vi "MGI Daemon Implementation.vi"(9 "Ignore Warnings? (F: Process Errors and Warnings)":bool, 10 "Log Dir":path, 11 "MGI Error Reporter Dialog In":refnum<class "MGI Error Reporter Dialog.lvclass">) -> (3 "MGI Error Reporter Out":refnum<class "MGI Error Reporter Dialog.lvclass">)   [LabVIEW 2016, in "MGI Error Reporter Dialog.lvclass"]
doc: "Implementation of the Error Handler Loop. This VI is separated from the Front Panel Controls so that the front panel control VI could be overridden in a child class and the appearance changed.\n\nAuthored by Shawn Walpole\nsupport@mooregoodideas.com\nwww.mooregoodideas.com\n\nCopyright (c) 2013, Moore Good Ideas, Inc.\n\nAll rights reserved.\n\nRedistribution and use in source and binary forms, with or without modification, are permitted provided that the following conditions are met:\n\n * Redistributions of source code must retain the above copyright notice, this list of conditions and the following disclaimer.\n * Redistributions in binary form must reproduce the above copyright notice, this list of conditions and the following disclaimer in the documentation and/or other materials provided with the distribution.\n * Neither the name of Moore Good Ideas, Inc. nor the names of its contributors may be used to endorse or promote products derived from this software without specific prior written permission.\n\nTHIS SOFTWARE IS PROVIDED BY THE COPYRIGHT HOLDERS AND CONTRIBUTORS \"AS IS\" AND ANY EXPRESS OR IMPLIED WARRANTIES, INCLUDING, BUT NOT LIMITED TO, THE IMPLIED WARRANTIES OF MERCHANTABILITY AND FITNESS FOR A PARTICULAR PURPOSE ARE DISCLAIMED. IN NO EVENT SHALL THE COPYRIGHT OWNER OR CONTRIBUTORS BE LIABLE FOR ANY DIRECT, INDIRECT, INCIDENTAL, SPECIAL, EXEMPLARY, OR CONSEQUENTIAL DAMAGES (INCLUDING, BUT NOT LIMITED TO, PROCUREMENT OF SUBSTITUTE GOODS OR SERVICES; LOSS OF USE, DATA, OR PROFITS; OR BUSINESS INTERRUPTION) HOWEVER CAUSED AND ON ANY THEORY OF LIABILITY, WHETHER IN CONTRACT, STRICT LIABILITY, OR TORT (INCLUDING NEGLIGENCE OR OTHERWISE) ARISING IN ANY WAY OUT OF THE USE OF THIS SOFTWARE, EVEN IF ADVISED OF THE POSSIBILITY OF SUCH DAMAGE."
uses:
  <userlib>/_MGI/Error Reporter/MGI Error Reporter Dialog/MGI Error Reporter Dialog.lvclass
  <userlib>/_MGI/Error Reporter/MGI Error Reporter Dialog/MGI Error Reporter Dialog.lvclass/MGI Error Reporter Dialog.ctl
  <vilib>/event_ctls.llb/sizeaction.ctl
  <vilib>/event_ctls.llb/panelstate.ctl
  <userlib>/_MGI/Error Reporter/MGI Error Reporter Dialog/Protected/MGI Control Enum.ctl
  <userlib>/_MGI/Error Reporter/MGI Error Reporter Dialog/MGI ERD LB Row Base/MGI ERD LB Row Base.lvclass
  <userlib>/_MGI/Error Reporter/MGI Error Reporter Base/MGI Error Reporter Base.lvclass
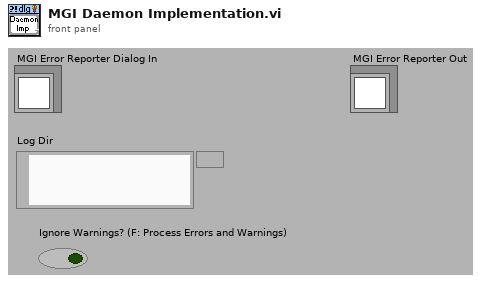
[diagram p1: front panel]
types:
  T1 = typedef "panelstate.ctl" = enum32{"Standard", "Minimized", "Maximized"}
  T2 = typedef "sizeaction.ctl" = enum32{"Minimized", "Maximized", "Resized"}
  T3 = typedef "LVRectTypeDef.ctl" = cluster{"Left":i16, "Top":i16, "Right":i16, "Bottom":i16}
  T4 = typedef "MGI Error Reporter Dialog.lvclass/MGI Control Enum.ctl" = enum16{"Error LB", "Details String", "Caller Ring", "Message String", "Clear Button"}
  T5 = typedef "LVPoint32TypeDef.ctl" = cluster{"Horizontal":i32, "Vertical":i32}
  T6 = typedef "MGI Error Reporter Dialog.lvclass/MGI Dialog UI Refs Cluster.ctl" = cluster{"LB Ref":refnum<vi>, "Details Ref":refnum<vi>, "Caller Ring Ref":refnum<vi>, "Message Ref":refnum<vi>, "Clear Btn Ref":refnum<vi>}
  T7 = typedef "MGI Error Reporter Base.lvclass/Cmd Enum.ctl" = enum16{"Quit", "Show UI"}
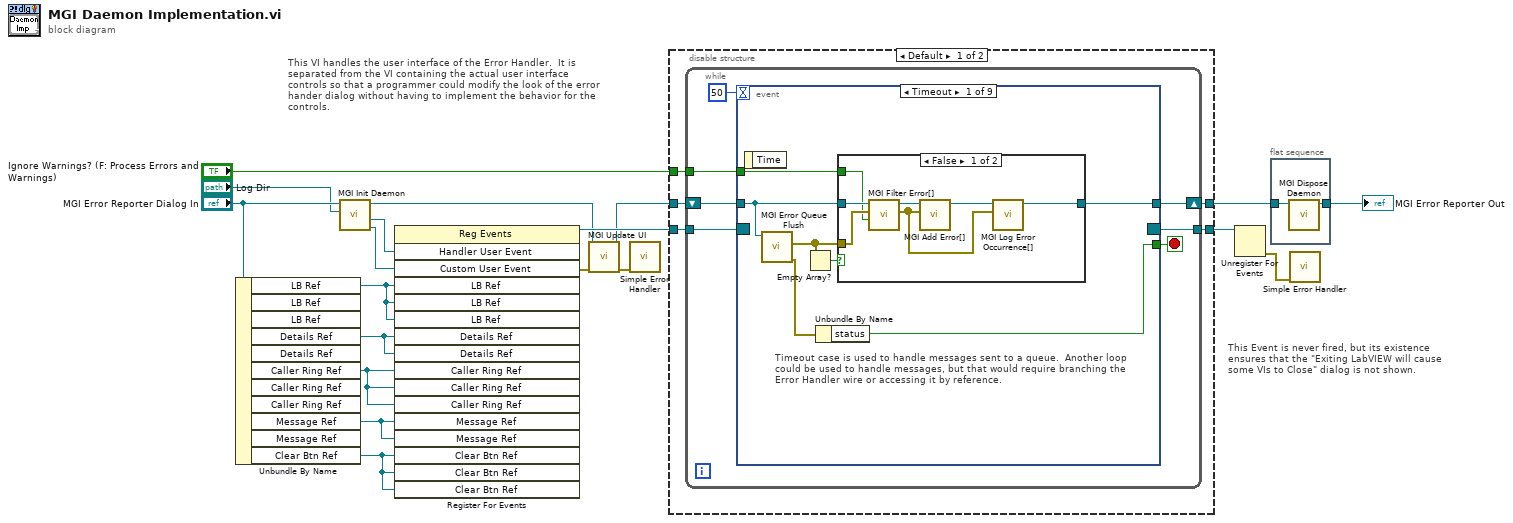
[diagram p0: block diagram]
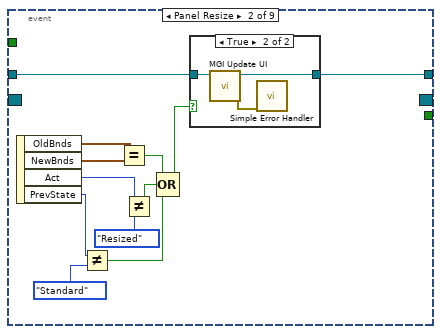
[diagram p3: hidden frame]
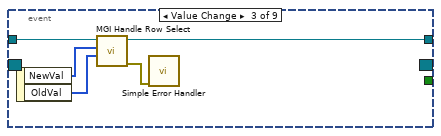
[diagram p5: hidden frame]
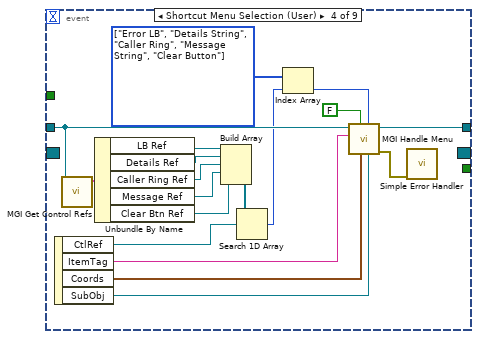
[diagram p6: hidden frame]
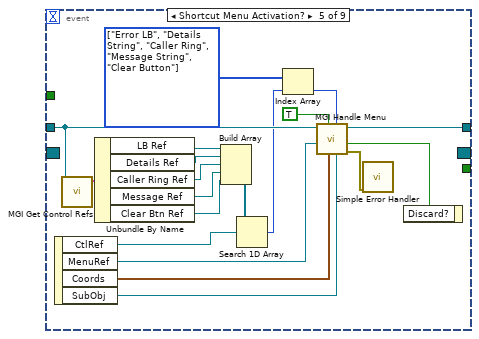
[diagram p7: hidden frame]
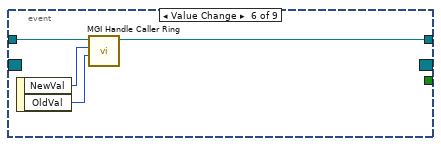
[diagram p8: hidden frame]
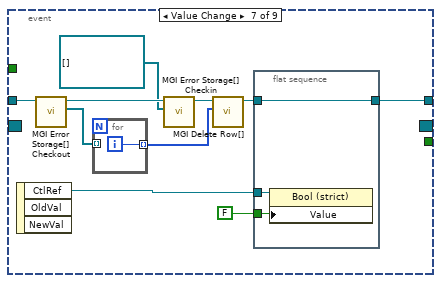
[diagram p9: hidden frame]
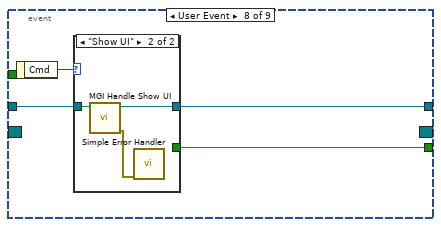
[diagram p10: hidden frame]
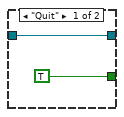
[diagram p11: hidden frame]
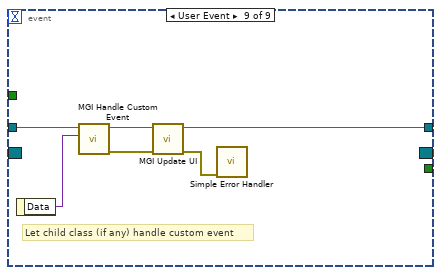
[diagram p12: hidden frame]
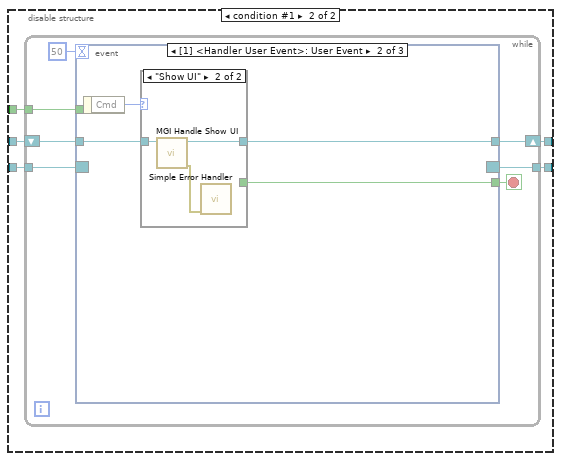
[diagram p13: hidden frame]
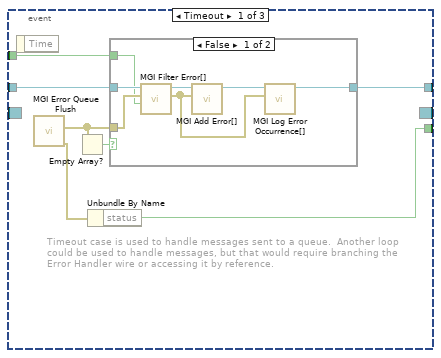
[diagram p14: hidden frame]
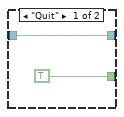
[diagram p16: hidden frame]
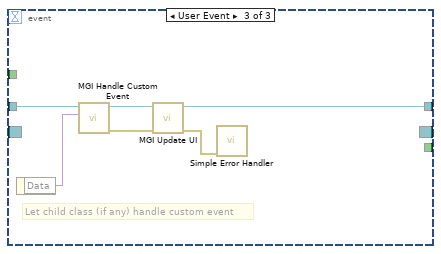
[diagram p17: hidden frame]
diagram:
  # "This Event is never fired, but its existence ensures that the \"Exiting LabVIEW will cause some VIs to Close\" dialog is not shown."
  # "This VI handles the user interface of the Error Handler.  It is separated from the VI containing the actual user interface controls so that a programmer could modify the look of the error hander dialog without having to implement the behavior for the controls."
  n1 = Unbundle By Name("MGI Error Reporter Dialog In") -> ("LB Ref"=w6:refnum<vi>, "Details Ref"=w5:refnum<vi>, "Caller Ring Ref"=w2:refnum<vi>, "Message Ref"=w8:refnum<vi>, "Clear Btn Ref"=w1:refnum<vi>)  [unwired: 6 out]
  n2 = call-dynamic "MGI Init Daemon.vi"("Err Dir"="Log Dir", "MGI Error Reporter Base In"="MGI Error Reporter Dialog In") -> ("Custom User Event"=w19:refnum<user-event>, "Handler User Event"=w18:refnum<user-event>, "MGI Error Reporter Base Out"=w11:refnum<class "MGI Error Reporter Dialog.lvclass">)  [unwired: 7 out]
  n3 = register-events(w18, w19, w6, w6, w6, w5, w5, w2, w2, w2, w8, w8, w1, w1, w1) -> (reference out=w17:refnum<event-registration>, error out=w13:errorcluster)  [unwired: 2 in]
  n4 = call-dynamic "MGI Update UI.vi"("error in (no error)"=w13, "MGI Error Handler in"=w11) -> ("error out"=w4:errorcluster, "MGI Error Handler out"=w14:refnum<class "MGI Error Reporter Dialog.lvclass">)  [unwired: 8 out]
  n5 = call <vilib>:"Simple Error Handler.vi"("error in (no error)"=w4) -> ()  [unwired: 1 in, 8 out]
  n6 = disable-structure shown="Default" {
    disable-tunnel: w17 -> [w24 w142]
    disable-tunnel: [w23 w141] -> w15
    disable-tunnel: w14 -> [w22 w140]
    disable-tunnel: [w21 w139] -> w12
    disable-tunnel: "Ignore Warnings? (F: Process Errors and Warnings)" -> [w20 w138]
    frame condition #0 (active) {
      n7 = while {
        tunnel: w24 -> [w25]
        shift-right: [w29] -> w23
        shift-left: w22 -> [w30]
        tunnel: [w27] -> w21
        tunnel: w20 -> [w26]
        stop <- w31 stop-if-true
        n8 = event shown="[0] Timeout" {
          selector: w25 -> [_ _ _ _ _ _ _ _ _]
          dyn-events: [_ _ _ _ _ _ _ _ _] -> w27
          timeout: 50 -> [_ _ _ _ _ _ _ _ _]
          tunnel: [w36 _ _ _ _ _ _ w123 _] -> w31
          tunnel: w30 -> [w32 w52 w67 w81 w101 w108 w113 w126 w137]
          tunnel: [w38 w51 w64 w79 w99 w107 w115 w125 w133] -> w29
          tunnel: w26 -> [w35 _ _ _ _ _ _ _ _]
          event Timeout {
            # "Timeout case is used to handle messages sent to a queue.  Another loop could be used to handle messages, but that would require branching the Error Handler wire or accessing it by reference."
            n9 = event-data() -> ()  [unwired: 2 out]
            n10 = call-dynamic "MGI Error Queue Flush.vi"("MGI Error Reporter Base In"=w32) -> ("error out"=w34:errorcluster, "Error[]"=w33:errorcluster[])  [unwired: 1 in, 8 out]
            n11 = Empty Array?(array=w33) -> (empty?=w37:bool)
            n12 = Unbundle By Name(w34) -> ("status"=w36:bool)
            n13 = case shown="False" w37 {
              tunnel: w32 -> [w44 w46]
              tunnel: [w39 w46] -> w38
              tunnel: w33 -> [w45 _]
              tunnel: w35 -> [w42 _]
              frame False {
                n14 = call-dynamic "MGI Filter Error[].vi"("Ignore Warnings? (F: Process Errors and Warnings)"=w42, "Error Occurence[]"=w45, "MGI Error Reporter Base in"=w44) -> ("Filtered Error[]"=w43:errorcluster[], "MGI Error Reporter Base out"=w41:refnum<class "MGI Error Reporter Dialog.lvclass">)  [unwired: 7 out]
                n15 = call-dynamic "MGI Add Error[].vi"("Error[]"=w43, "MGI Error Handler in"=w41) -> ("MGI Error Handler out"=w40:refnum<class "MGI Error Reporter Dialog.lvclass">)  [unwired: 1 in, 8 out]
                n16 = call-dynamic "MGI Log Error Occurrence[].vi"("Error Occurence[]"=w43, "MGI Error Reporter Base in"=w40) -> ("MGI Error Reporter Base out"=w39:refnum<class "MGI Error Reporter Dialog.lvclass">)  [unwired: 2 in, 7 out]
              }
              frame True {
              }
            }
          }
          event Panel Resize {
            n17 = event-data() -> ("OldBnds"=w58:T3, "NewBnds"=w57:T3, "Act"=w55:T2, "PrevState"=w49:T1)  [unwired: 1 out]
            n18 = Not Equal?(x=w49, y=panelstate."Standard" ("PrevState")) -> (x != y?=w47:bool)
            n19 = Equal?(x=w58, y=w57) -> (x = y?=w56:bool)
            n20 = Not Equal?(x=w55, y=sizeaction."Resized" ("Act")) -> (x != y?=w53:bool)
            n21 = Compound Arithmetic op=OR(w56, w53, w47) -> (w50:bool)
            n22 = case shown="True" w50 {
              tunnel: w52 -> [w59 w62]
              tunnel: [w59 w61] -> w51
              frame False {
              }
              frame True {
                n23 = call-dynamic "MGI Update UI.vi"("MGI Error Handler in"=w62) -> ("error out"=w60:errorcluster, "MGI Error Handler out"=w61:refnum<class "MGI Error Reporter Dialog.lvclass">)  [unwired: 1 in, 8 out]
                n24 = call <vilib>:"Simple Error Handler.vi"("error in (no error)"=w60) -> ()  [unwired: 1 in, 8 out]
              }
            }
          }
          event Value Change {
            n25 = event-data() -> ("NewVal"=w66:i32[], "OldVal"=w65:i32[])  [unwired: 1 out]
            n26 = call-dynamic "MGI Handle Row Select.vi"("Old Selected[]"=w65, "Selected[]"=w66, "MGI Error Handler in"=w67) -> ("error out"=w63:errorcluster, "MGI Error Handler out"=w64:refnum<class "MGI Error Reporter Dialog.lvclass">)  [unwired: 1 in, 6 out]
            n27 = call <vilib>:"Simple Error Handler.vi"("error in (no error)"=w63) -> ()  [unwired: 1 in, 8 out]
          }
          event Shortcut Menu Selection (User) {
            w72 = T4[] [enum."Error LB", enum."Details String", enum."Caller Ring", enum."Message String", enum."Clear Button"] items=["Error LB", "Details String", "Caller Ring", "Message String", "Clear Button"]
            n28 = event-data() -> ("CtlRef"=w73:refnum<vi>, "ItemTag"=w85:string, "Coords"=w83:T5, "SubObj"=w82:refnum<vi>)  [unwired: 1 out]
            n29 = call <userlib>:"MGI Get Control Refs.vi"("MGI Error Dialog.lvclass"=w81) -> ("Refs"=w80:T6)  [unwired: 10 out]
            n30 = Unbundle By Name(w80) -> ("LB Ref"=w78:refnum<vi>, "Details Ref"=w77:refnum<vi>, "Caller Ring Ref"=w76:refnum<vi>, "Message Ref"=w75:refnum<vi>, "Clear Btn Ref"=w68:refnum<vi>)
            n31 = Build Array(w78, w77, w76, w75, w68) -> (w74:refnum<vi>[])
            n32 = Search 1D Array(1D array=w74, element=w73) -> (index of element=w71:i32)  [unwired: 1 out]
            n33 = Index Array(array=w72, index=w71) -> (element=w70:T4)
            n34 = call-dynamic "MGI Handle Menu.vi"("SubObj"=w82, "Control Enum"=w70, "Coord"=w83, "Activation? (F:Selection)"=FALSE, "Selection:Menu Tag"=w85, "MGI Error Reporter Dialog"=w81) -> ("error out"=w69:errorcluster, "MGI Error Reporter Dialog Out"=w79:refnum<class "MGI Error Reporter Dialog.lvclass">)  [unwired: 2 in, 2 out]
            n35 = call <vilib>:"Simple Error Handler.vi"("error in (no error)"=w69) -> ()  [unwired: 1 in, 8 out]
          }
          event Shortcut Menu Activation? {
            w92 = T4[] [enum."Error LB", enum."Details String", enum."Caller Ring", enum."Message String", enum."Clear Button"] items=["Error LB", "Details String", "Caller Ring", "Message String", "Clear Button"]
            n36 = event-data() -> ("CtlRef"=w93:refnum<vi>, "MenuRef"=w89:refnum<k9>, "Coords"=w103:T5, "SubObj"=w102:refnum<vi>)  [unwired: 1 out]
            n37 = call <userlib>:"MGI Get Control Refs.vi"("MGI Error Dialog.lvclass"=w101) -> ("Refs"=w100:T6)  [unwired: 10 out]
            n38 = Unbundle By Name(w100) -> ("LB Ref"=w98:refnum<vi>, "Details Ref"=w97:refnum<vi>, "Caller Ring Ref"=w96:refnum<vi>, "Message Ref"=w95:refnum<vi>, "Clear Btn Ref"=w86:refnum<vi>)
            n39 = Build Array(w98, w97, w96, w95, w86) -> (w94:refnum<vi>[])
            n40 = Search 1D Array(1D array=w94, element=w93) -> (index of element=w91:i32)  [unwired: 1 out]
            n41 = Index Array(array=w92, index=w91) -> (element=w90:T4)
            n42 = call-dynamic "MGI Handle Menu.vi"("SubObj"=w102, "Control Enum"=w90, "Coord"=w103, "Activation? (F:Selection)"=TRUE, "Activation:MenuRef"=w89, "MGI Error Reporter Dialog"=w101) -> ("error out"=w87:errorcluster, "Activation:Discard?"=w88:bool, "MGI Error Reporter Dialog Out"=w99:refnum<class "MGI Error Reporter Dialog.lvclass">)  [unwired: 2 in, 1 out]
            n43 = call <vilib>:"Simple Error Handler.vi"("error in (no error)"=w87) -> ()  [unwired: 1 in, 8 out]
            n44 = event-data("Discard?"=w88) -> ()  [unwired: 1 in, 1 out]
          }
          event Value Change {
            n45 = event-data() -> ("NewVal"=w106:u16, "OldVal"=w105:u16)  [unwired: 1 out]
            n46 = call-dynamic "MGI Handle Caller Ring.vi"("Old Value"=w105, "New Value"=w106, "MGI Error Reporter Dialog in"=w108) -> ("MGI Error Reporter Dialog out"=w107:refnum<class "MGI Error Reporter Dialog.lvclass">)  [unwired: 1 in, 7 out]
          }
          event Value Change {
            n47 = event-data() -> ("CtlRef"=w117:refnum<vi>)  [unwired: 3 out]
            n48 = call <userlib>:"MGI Error Storage[] Checkout.vi"("MGI Error Reporter Dialog In"=w113) -> ("ErrStorage[row]"=w112:refnum<class "MGI ERD LB Row Base.lvclass">[], "MGI Error Reporter Dialog Out"=w111:refnum<class "MGI Error Reporter Dialog.lvclass">)  [unwired: 9 out]
            n49 = for {
              tunnel: w112 -> [_] mode=indexing
              tunnel: [w122] -> w118 mode=indexing
              i -> [w122]
            }
            n50 = call <userlib>:"MGI Error Storage[] Checkin.vi"("ErrStorage[row]"=refnum<class "MGI ERD LB Row Base.lvclass">[] [], "MGI Error Reporter Dialog In"=w111) -> ("MGI Error Reporter Dialog Out"=w110:refnum<class "MGI Error Reporter Dialog.lvclass">)  [unwired: 9 out]
            n51 = call-dynamic "MGI Delete Row[].vi"("Listbox row[] to delete"=w118, "MGI Error Handler in"=w110) -> ("MGI Error Handler out"=w116:refnum<class "MGI Error Reporter Dialog.lvclass">)  [unwired: 1 in, 8 out]
            n52 = flat-sequence {
              tunnel: w117 -> [w121]
              tunnel: w116 -> [w120]
              tunnel: [w120] -> w115
              tunnel: FALSE -> [w119]
              frame #0 {
                n53 = property class="Bool (strict)"(reference=w121, "Value"=w119) -> ()  [unwired: 1 in, 2 out]
              }
            }
          }
          event User Event {
            n54 = event-data() -> ("Cmd"=w124:T7)  [unwired: 1 out]
            n55 = case shown="\"Show UI\"" w124 {
              tunnel: w126 -> [w128 w131]
              tunnel: [w128 w130] -> w125
              tunnel: [TRUE _] -> w123
              frame "Quit" {
              }
              frame "Show UI" {
                n56 = call-dynamic "MGI Handle Show UI.vi"("MGI Error Reporter Dialog In"=w131) -> ("error out"=w129:errorcluster, "MGI Error Reporter Dialog Out"=w130:refnum<class "MGI Error Reporter Dialog.lvclass">)  [unwired: 3 in, 6 out]
                n57 = call <vilib>:"Simple Error Handler.vi"("error in (no error)"=w129) -> ()  [unwired: 1 in, 8 out]
              }
            }
          }
          event User Event {
            # "Let child class (if any) handle custom event"
            n58 = event-data() -> ("Data"=w136:variant)  [unwired: 1 out]
            n59 = call-dynamic "MGI Handle Custom Event.vi"("Data"=w136, "MGI Error Reporter Base In"=w137) -> ("error out"=w134:errorcluster, "MGI Error Reporter Base In"=w135:refnum<class "MGI Error Reporter Dialog.lvclass">)  [unwired: 1 in, 7 out]
            n60 = call-dynamic "MGI Update UI.vi"("error in (no error)"=w134, "MGI Error Handler in"=w135) -> ("error out"=w132:errorcluster, "MGI Error Handler out"=w133:refnum<class "MGI Error Reporter Dialog.lvclass">)  [unwired: 8 out]
            n61 = call <vilib>:"Simple Error Handler.vi"("error in (no error)"=w132) -> ()  [unwired: 1 in, 8 out]
          }
        }
      }
    }
    frame condition #1 {
      n62 = while {
        tunnel: w142 -> [w144]
        shift-right: [w147] -> w141
        shift-left: w140 -> [w148]
        tunnel: [w146] -> w139
        tunnel: w138 -> [w145]
        stop <- w149 stop-if-true
        n63 = event shown="[1] <Handler User Event>: User Event" {
          selector: w144 -> [_ _ _]
          dyn-events: [_ _ _] -> w146
          timeout: 50 -> [_ _ _]
          tunnel: [w153 w165 _] -> w149
          tunnel: w148 -> [w156 w168 w179]
          tunnel: [w155 w167 w175] -> w147
          tunnel: w145 -> [w152 _ _]
          event Timeout {
            # "Timeout case is used to handle messages sent to a queue.  Another loop could be used to handle messages, but that would require branching the Error Handler wire or accessing it by reference."
            n64 = event-data() -> ()  [unwired: 1 in, 1 out]
            n65 = call-dynamic "MGI Error Queue Flush.vi"() -> ("error out"=w151:errorcluster, "Error[]"=w150:errorcluster[])  [unwired: 10 in]
            n66 = Empty Array?(array=w150) -> (empty?=w154:bool)
            n67 = Unbundle By Name(w151) -> ("status"=w153:bool)
            n68 = case shown="False" w154 {
              tunnel: w156 -> [w162 w164]
              tunnel: [w157 w164] -> w155
              tunnel: w150 -> [w163 _]
              tunnel: w152 -> [w160 _]
              frame False {
                n69 = call-dynamic "MGI Filter Error[].vi"("Ignore Warnings? (F: Process Errors and Warnings)"=w160, "Error Occurence[]"=w163, "MGI Error Reporter Base in"=w162) -> ("Filtered Error[]"=w161:errorcluster[], "MGI Error Reporter Base out"=w159:refnum<class "MGI Error Reporter Dialog.lvclass">)  [unwired: 7 in]
                n70 = call-dynamic "MGI Add Error[].vi"("Error[]"=w161, "MGI Error Handler in"=w159) -> ("MGI Error Handler out"=w158:refnum<class "MGI Error Reporter Dialog.lvclass">)  [unwired: 8 in, 1 out]
                n71 = call-dynamic "MGI Log Error Occurrence[].vi"("Error Occurence[]"=w161, "MGI Error Reporter Base in"=w158) -> ("MGI Error Reporter Base out"=w157:refnum<class "MGI Error Reporter Dialog.lvclass">)  [unwired: 8 in, 1 out]
              }
              frame True {
              }
            }
          }
          event User Event {
            n72 = event-data() -> ("Cmd"=w166:T7)  [unwired: 1 in]
            n73 = case shown="\"Show UI\"" w166 {
              tunnel: w168 -> [w170 w173]
              tunnel: [w170 w172] -> w167
              tunnel: [TRUE _] -> w165
              frame "Quit" {
              }
              frame "Show UI" {
                n74 = call-dynamic "MGI Handle Show UI.vi"("MGI Error Reporter Dialog In"=w173) -> ("error out"=w171:errorcluster, "MGI Error Reporter Dialog Out"=w172:refnum<class "MGI Error Reporter Dialog.lvclass">)  [unwired: 9 in]
                n75 = call <vilib>:"Simple Error Handler.vi"("error in (no error)"=w171) -> ()  [unwired: 4 in, 5 out]
              }
            }
          }
          event User Event {
            # "Let child class (if any) handle custom event"
            n76 = event-data() -> ("Data"=w178:variant)  [unwired: 1 in]
            n77 = call-dynamic "MGI Handle Custom Event.vi"("Data"=w178, "MGI Error Reporter Base In"=w179) -> ("error out"=w176:errorcluster, "MGI Error Reporter Base In"=w177:refnum<class "MGI Error Reporter Dialog.lvclass">)  [unwired: 8 in]
            n78 = call-dynamic "MGI Update UI.vi"("error in (no error)"=w176, "MGI Error Handler in"=w177) -> ("error out"=w174:errorcluster, "MGI Error Handler out"=w175:refnum<class "MGI Error Reporter Dialog.lvclass">)  [unwired: 8 in]
            n79 = call <vilib>:"Simple Error Handler.vi"("error in (no error)"=w174) -> ()  [unwired: 4 in, 5 out]
          }
        }
      }
    }
  }
  n80 = Unregister For Events(event registration refnum=w12) -> (error out=w3:errorcluster)  [unwired: 1 in]
  n81 = flat-sequence {
    tunnel: [w181] -> w16
    tunnel: w15 -> [w180]
    frame #0 {
      n82 = call-dynamic "MGI Dispose Daemon.vi"("MGI Error Reporter Base In"=w180) -> ("MGI Error Reporter Base Out"=w181:refnum<class "MGI Error Reporter Dialog.lvclass">)  [unwired: 10 out]
    }
  }
  n83 = call <vilib>:"Simple Error Handler.vi"("error in (no error)"=w3) -> ()  [unwired: 1 in, 8 out]
  "MGI Error Reporter Out" <- w16
